vi "Transistor_Characteristics_NikhilSanga_Dipto_Group4.vi"() -> ()   [LabVIEW 2020]
panel:
  in  "?":T1(tab)
  in  "stop":bool caption="Stop Button"
  out "Transistor Static Characteristics":cluster{dbl[], dbl[]}[](graph)
  in  "Start Button":bool
  out "Temperature / °C":dbl
  out "UB /V":dbl format="%#_3g"
  out "UBE /V":dbl format="%#_3g"
  out "IB /mA":dbl format="%#_3g"
  out "UCE  /V":dbl format="%#_3g"
  out "UC /V":dbl format="%#_3g"
  out "IC /mA":dbl format="%#_3g"
  # "Output Characteristics of Bipolar Transistor (BC547)"
  # "Version : 20.0"
  # "Output Characteristics of Bipolar Transistor (BC547)"
  # "Current Monitoring"
  # "Voltage Monitoring"
  # "Temperature Monitoring"
  # "Version : 20.0"
  # "Output Characteristics of Bipolar Transistor (BC547)"
  # "Guided by:\nProf. Dr. -Ing. Friedrich Fleischmann\nDipl.-Ing. René Ramson\n\nPresented By:\nNikhil Shrikrishna Sanga - 5366338\nMd Shahriar Dipto           - 5227587"
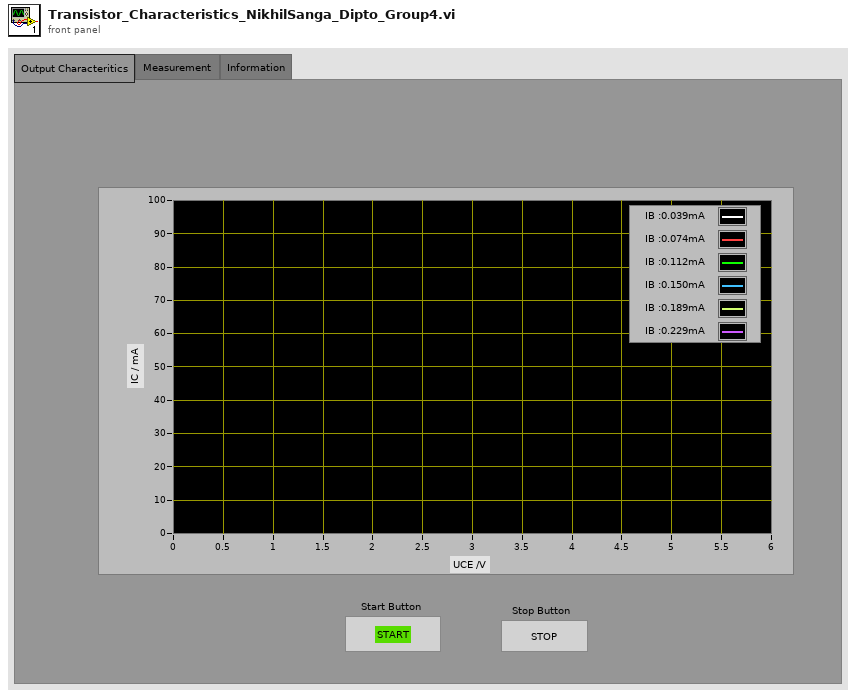
[diagram p1: front panel]
types:
  T1 = enum32{"Output Characteritics", "Measurement ", "Information"}
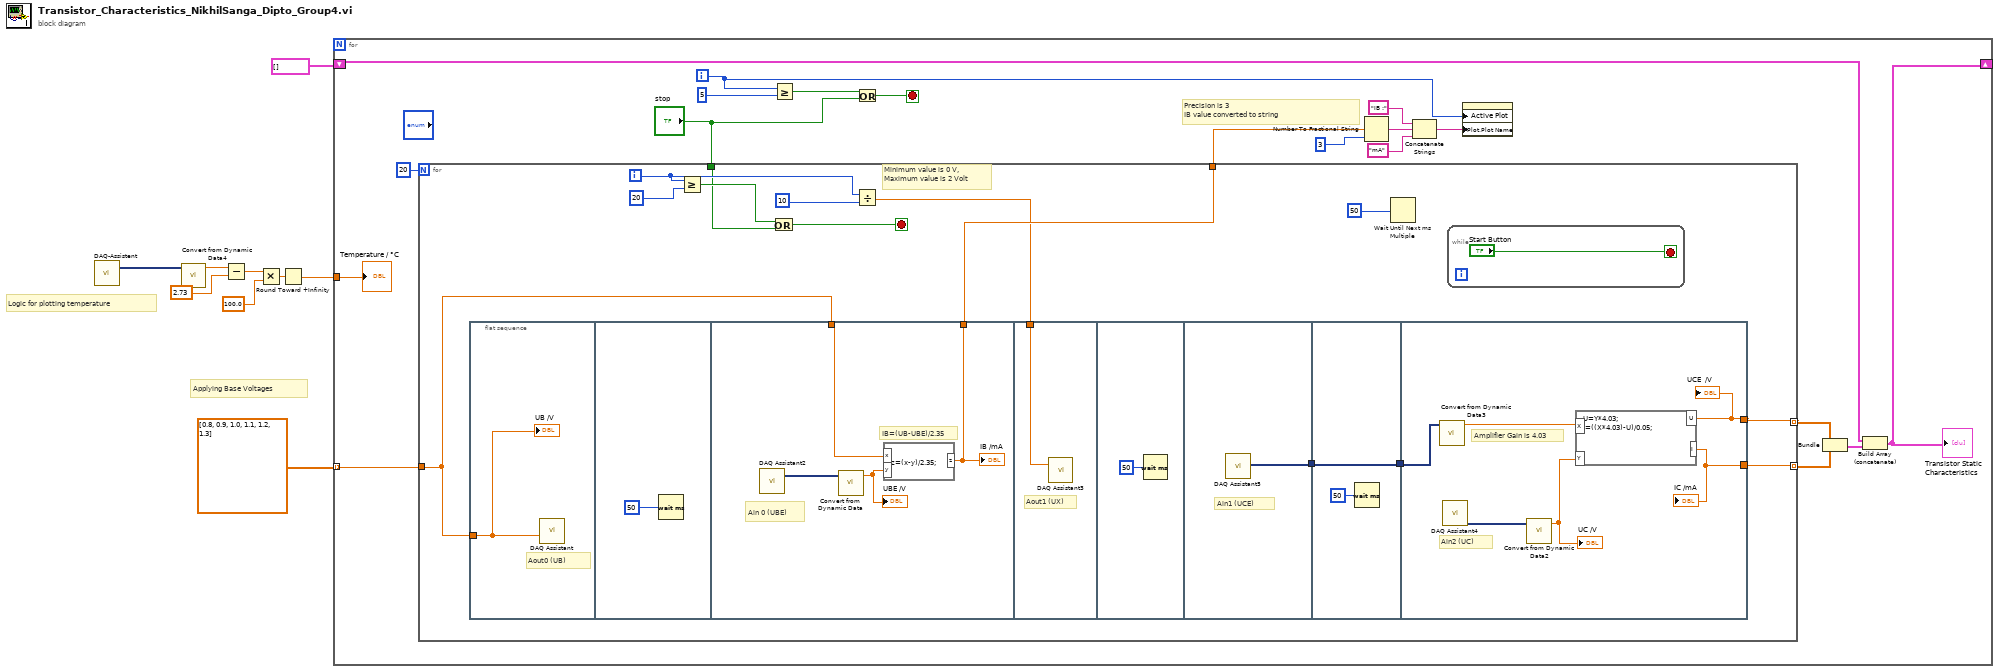
[diagram p0: block diagram]
diagram:
  # "Logic for plotting temperature"
  # "Applying Base Voltages"
  n1 = call "DAQ-Assistent"() -> ("data"=w7:dynamicdata)  [unwired: 17 in, 2 out]
  n2 = call "Convert from Dynamic Data4"("Dynamic Data Type"=w7) -> ("Scalar"=w6:dbl)  [unwired: 1 in, 2 out]
  n3 = Subtract(x=w6, y=2.73) -> (x-y=w4:dbl)
  n4 = Multiply(x=w4, y=100.0) -> (x*y=w2:dbl)
  n5 = Round Toward +Infinity(x=w2) -> (ceil(x): smallest int >= x=w1:dbl)
  n6 = for {
    shift-right: [w14] -> _
    shift-left: cluster{dbl[], dbl[]}[] [] -> [w12]
    tunnel: dbl[] [0.8, 0.9, 1.0, 1.1, 1.2, 1.3] ("Array") -> [w11] mode=indexing
    tunnel: w1 -> [w10]
    i -> [w15]
    stop <- w16 stop-if-true
    # "Precision is 3 \nIB value converted to string"
    n7 = for {
      N: 20 -> [_]
      tunnel: [w38] -> w27 mode=indexing
      tunnel: [w37] -> w28 mode=indexing
      tunnel: [w39] -> w25
      tunnel: "stop" -> [w31]
      tunnel: w11 -> [w30]
      i -> [w35]
      stop <- w29 stop-if-true
      # "Minimum value is 0 V,\nMaximum value is 2 Volt"
      n8 = flat-sequence {
        tunnel: w30 -> [w44]
        tunnel: [w46] -> w39
        tunnel: w30 -> [w48]
        tunnel: w36 -> [w50]
        tunnel: [w52] -> w34
        tunnel: w34 -> [w54]
        tunnel: [w54] -> w33
        tunnel: w33 -> [w56]
        tunnel: [w60] -> w38
        tunnel: [w59] -> w37
        frame #0 {
          # "Aout0 (UB)"
          n9 = call "DAQ Assistant"("data"=w44) -> ()  [unwired: 17 in, 2 out]
          "UB /V" <- w44
        }
        frame #1 {
          n10 = Wait (ms)(milliseconds to wait=u32 50) -> ()  [unwired: 1 out]
        }
        frame #2 {
          # "Ain 0 (UBE)"
          # "IB=(UB-UBE)/2.35"
          n11 = call "DAQ Assistant2"() -> ("data"=w49:dynamicdata)  [unwired: 17 in, 2 out]
          n12 = call "Convert from Dynamic Data"("Dynamic Data Type"=w49) -> ("Scalar"=w47:dbl)  [unwired: 3 in]
          "UBE /V" <- w47
          n13 = formula code="z=(x-y)/2.35;"("x"=w48, "y"=w47) -> ("z"=w46:dbl)
          "IB /mA" <- w46
        }
        frame #3 {
          # "Aout1 (UX)"
          n14 = call "DAQ Assistant3"("data"=w50) -> ()  [unwired: 17 in, 2 out]
        }
        frame #4 {
          n15 = Wait (ms)(milliseconds to wait=u32 50) -> ()  [unwired: 1 out]
        }
        frame #5 {
          # "Ain1 (UCE)"
          n16 = call "DAQ Assistant5"() -> ("data"=w52:dynamicdata)  [unwired: 17 in, 2 out]
        }
        frame #6 {
          n17 = Wait (ms)(milliseconds to wait=u32 50) -> ()  [unwired: 1 out]
        }
        frame #7 {
          # "Amplifier Gain is 4.03"
          # "Ain2 (UC)"
          n18 = call "Convert from Dynamic Data3"("Dynamic Data Type"=w56) -> ("Scalar"=w57:dbl)  [unwired: 3 in]
          n19 = call "DAQ Assistant4"() -> ("data"=w58:dynamicdata)  [unwired: 17 in, 2 out]
          n20 = call "Convert from Dynamic Data2"("Dynamic Data Type"=w58) -> ("Scalar"=w55:dbl)  [unwired: 3 in]
          "UC /V" <- w55
          n21 = formula code="U=Y*4.03;\nI=((X*4.03)-U)/0.05;"("X"=w57, "Y"=w55) -> ("I"=w59:dbl, "U"=w60:dbl)
          "UCE  /V" <- w60
          "IC /mA" <- w59
        }
      }
      n22 = Greater Or Equal?(x=w35, y=20) -> (x >= y?=w32:bool)
      n23 = Or(x=w32, y=w31) -> (x .or. y?=w29:bool)
      n24 = Divide(x=w35, y=10) -> (x/y=w36:dbl)
      n25 = Wait Until Next ms Multiple(millisecond multiple=u32 50) -> ()  [unwired: 1 out]
      n26 = while {
        stop <- "Start Button" stop-if-true
      }
    }
    n27 = Greater Or Equal?(x=w15, y=5) -> (x >= y?=w18:bool)
    n28 = Or(x=w18, y="stop") -> (x .or. y?=w16:bool)
    n29 = Number To Fractional String(number=w25, precision (6)=i16 3) -> (F-format string=w24:string)  [unwired: 2 in]
    n30 = Concatenate Strings("IB :" ("string"), w24, "mA" ("string")) -> (w21:string)
    n31 = property on="Transistor Static Characteristics" class="XYGraph (strict)"("Active Plot"=w15, "Plot.Plot Name"=w21) -> ()  [unwired: 2 in, 2 out]
    n32 = Bundle(w27, w28) -> (w13:cluster{dbl[], dbl[]})  [unwired: 1 in]
    n33 = Build Array (concatenate)(w12, w13) -> (w14:cluster{dbl[], dbl[]}[])
    "Transistor Static Characteristics" <- w14
    "Temperature / °C" <- w10
  }
